vi "CameraList.vi"(0 "error in":errorcluster, 3 "node":string) -> (1 "error out":errorcluster, 4 "Cameras List":T1)   [LabVIEW 2015]
doc: "Lists cameras currently open.\n\nIf you are running 1.1.0 or higher, you will only see two cameras powered on. This is a new feature of ROS Indigo. To open another camera, first close one that is currently open."
uses:
  ROS/Code/Console/Servers/ServerSubs/TopicDef.ctl
  ROS/Code/SubVIs/_ROSDirection.ctl
panel:
  out "Reply":string
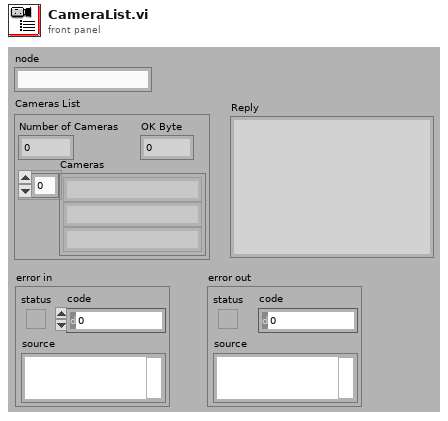
[diagram p1: front panel]
types:
  T1 = cluster{"Number of Cameras":i32, "Cameras":string[], "OK Byte":u8}
  T2 = typedef "TopicDef.ctl" = cluster{"Topic":string, "Type":string, "Action":T3, "Update (ms)":u16, "queue size":u16}
  T3 = typedef "_ROSDirection.ctl" = enum16{"Node", "Publisher", "Subscriber", "ServiceClient", "ServiceProvider"}
  T4 = typedef "_ROSControl.ctl" = cluster{"topic port":u16, "Node":string, "topic":string, "type":string, "node port":u16, "error ":errorcluster, "Direction":T3, "Update (ms)":u16, "FIFO size":u16}
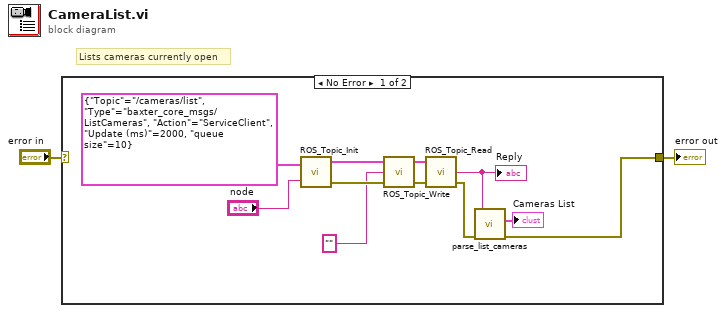
[diagram p0: block diagram]
diagram:
  # "Lists cameras currently open"
  n1 = case shown="No Error" "error in" {
    selector: "error in" -> [_ w14]
    tunnel: [w3 w14] -> w2
    frame No Error {
      n2 = call "ROS_Topic_Init.vi"("Definitions"=T2 {"Topic"="/cameras/list", "Type"="baxter_core_msgs/ListCameras", "Action"=enum."ServiceClient", "Update (ms)"=2000, "queue size"=10}, "node"="node") -> ("ROS out"=w12:T4, "error out"=w7:errorcluster)  [unwired: 1 in]
      n3 = call "ROS_Topic_Write.vi"("error in (no error)"=w7, "Msg in"="", "ROS in"=w12) -> ("error out"=w5:errorcluster, "ROS out"=w11:T4)  [unwired: 1 in]
      n4 = call "ROS_Topic_Read.vi"("error in (no error)"=w5, "ROS in"=w11) -> ("error out"=w4:errorcluster, "Reply"=w10:string)  [unwired: 1 in, 1 out]
      "Reply" <- w10
      n5 = call "parse_list_cameras.vi"("error in"=w4, "msg in"=w10) -> ("error out"=w3:errorcluster, "Cameras List"=→"Cameras List":T1)  [unwired: 3 in, 1 out]
    }
    frame Error {
    }
  }
  "error out" <- w2
